vi "SENS_FOM_RANG_COUP.vi"(0 "VISA IN":refnum<visa-resource-name>, 1 "Range number":i32, 2 "Couple Range to Primary Range ON/OFF":bool, 5 "error in":errorcluster, 7 "Channel":i32) -> (14 "VISA Out":refnum<visa-resource-name>, 19 "error out":errorcluster)   [LabVIEW 2018, in "PNA-X.lvlib"]
doc: "SENSe<cnum>:FOM:RANGe<n>:COUPled <bool> \n(Read-Write) Sets and returns the state of coupling (ON or OFF) of the specified range to the primary range. \nParameters \n<cnum> Any existing channel number; if unspecified, value is set to 1. \n<n> Range number to couple to primary range. An error is returned when attempting to \ncouple to the Primary range (1). \n<bool> ON (or 1) - Couple range to primary range. \nOFF (or 0) - Do NOT couple to primary range. \nExamples SENS:FOM:RANG:COUP 1 \nsense2:fom:range2:coupled 0 \nQuery Syntax SENSe<cnum>:FOM:RANGe<n>:COUPled? \nReturn Type Boolean \nDefault ON (or 1) Coupled \n1738"
uses:
  PNA-X.lvlib
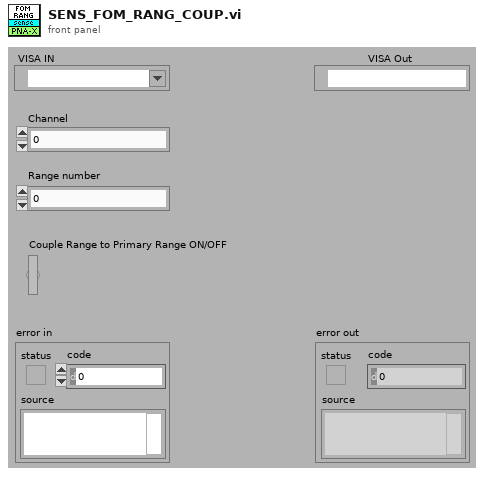
[diagram p1: front panel]
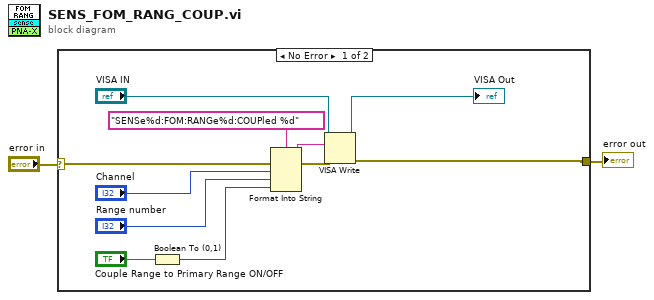
[diagram p0: block diagram]
diagram:
  n1 = case shown="No Error" "error in" {
    selector: "error in" -> [w13 w14]
    tunnel: [w8 w14] -> w1
    frame No Error {
      n2 = Boolean To (0,1)(Boolean="Couple Range to Primary Range ON/OFF") -> (0, 1=w3:i16)
      n3 = Format Into String(format string="SENSe%d:FOM:RANGe%d:COUPled %d" ("Cmdline"), error in=w13, "Channel", "Range number", w3) -> (resulting string=w11:string, error out=w12:errorcluster)  [unwired: 1 in]
      n4 = VISA Write(VISA resource name="VISA IN", write buffer=w11, error in (no error)=w12) -> (VISA resource name out=→"VISA Out":refnum<visa-resource-name>, error out=w8:errorcluster)  [unwired: 1 out]
    }
    frame Error {
    }
  }
  "error out" <- w1
